vi "Cascade.vi"(0 "LV MDI in":refnum<class "LV MDI.lvclass">, 5 "Order":T1=2 items=["List order"=2, "Z order"=4], 11 "error in (no error)":errorcluster) -> (4 "LV MDI out":refnum<class "LV MDI.lvclass">, 15 "error out":errorcluster)   [LabVIEW 2016, in "LV MDI.lvclass"]
doc: "Cascade child windows in MDI panel"
uses:
  LV MDI.lvclass
  Typedef/Cascade Order.ctl
  LV MDI.lvclass/LV MDI.ctl
  property/Read Parent Hwnd.vi
  property/Read Child Count.vi
  Document/Document base/Document.lvclass
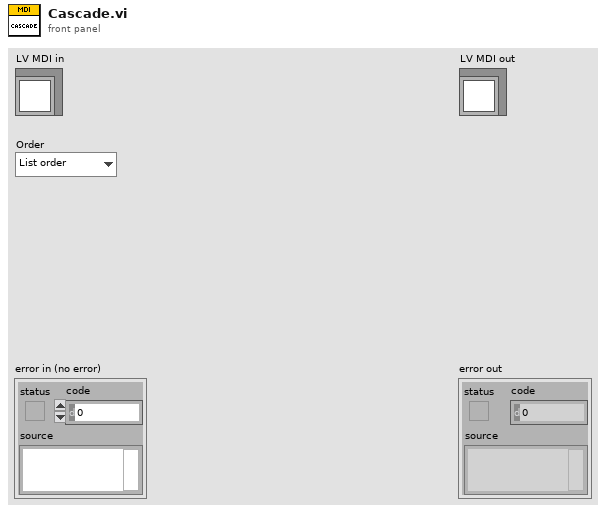
[diagram p1: front panel]
types:
  T1 = typedef "LV MDI.lvclass/Cascade Order.ctl" = u16
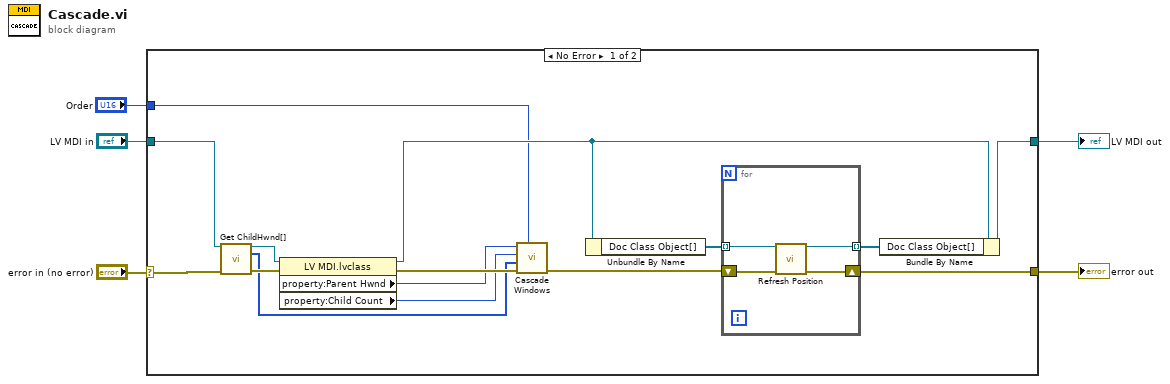
[diagram p0: block diagram]
diagram:
  n1 = case shown="No Error" "error in (no error)" {
    selector: "error in (no error)" -> [w20 w26]
    tunnel: [w14 w26] -> w4
    tunnel: [w10 w25] -> w2
    tunnel: "LV MDI in" -> [w19 w25]
    tunnel: "Order" -> [w9 _]
    frame No Error {
      n2 = call "Get ChildHwnd[].vi"("LV MDI in"=w19, "error in (no error)"=w20) -> ("LV MDI out"=w17:refnum<class "LV MDI.lvclass">, "ChildHwnd[]"=w8:u32[], "error out"=w18:errorcluster)  [unwired: 11 in]
      n3 = property class="LV MDI.lvclass"(reference=w17, error in=w18) -> (reference out=w11:refnum<class "LV MDI.lvclass">, error out=w16:errorcluster, "property:Parent Hwnd"=w7:i32, "property:Child Count"=w6:i32)
      n4 = call "Cascade Windows.vi"("Order"=w9, "error in (no error)"=w16, "ChildHwnd[]"=w8, "Child Count"=w6, "Parent Hwnd"=w7) -> ("error out"=w15:errorcluster)  [unwired: 6 in]
      n5 = Unbundle By Name(w11) -> ("Doc Class Object[]"=w13:refnum<class "Document.lvclass">[])
      n6 = for {
        shift-right: [w23] -> w14
        shift-left: w15 -> [w24]
        tunnel: w13 -> [w22] mode=indexing
        tunnel: [w21] -> w12 mode=indexing
        n7 = call-dynamic "Refresh Position.vi"("Document in"=w22, "error in (no error)"=w24) -> ("Document out"=w21:refnum<class "Document.lvclass">, "error out"=w23:errorcluster)  [unwired: 12 in]
      }
      n8 = Bundle By Name(cluster=w11, "Doc Class Object[]"=w12) -> (w10:refnum<class "LV MDI.lvclass">)
    }
    frame Error {
    }
  }
  "error out" <- w4
  "LV MDI out" <- w2
